vi "ReadFilesInFolder.vi"(7 "Numeric":i32, 8 "error in (no error)":errorcluster, 9 "Read entire Folder":bool, 10 "path":path, 11 "Path in":refnum<vi>) -> (0 "error out":errorcluster, 2 "t":i32, 3 "filenames":string[](array[string]))   [LabVIEW 2020]
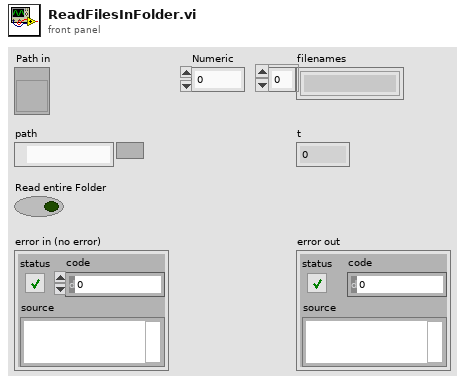
[diagram p1: front panel]
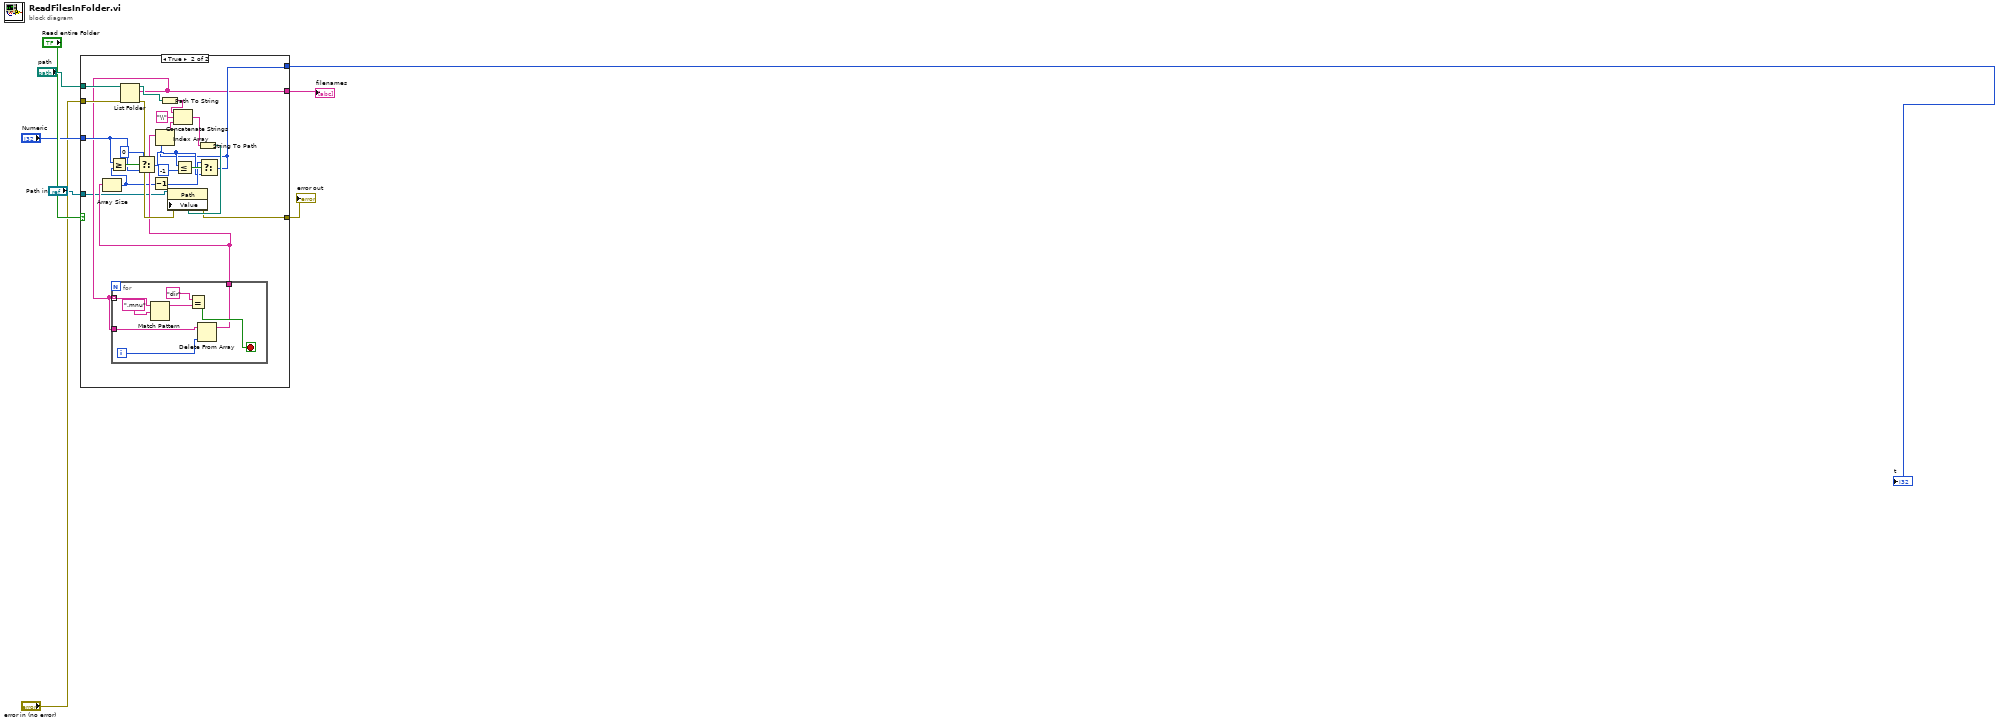
[diagram p0: block diagram]
diagram:
  n1 = case shown="True" "Read entire Folder" {
    tunnel: "error in (no error)" -> [w9 w26]
    tunnel: "Numeric" -> [w10 w24]
    tunnel: [w10 w15] -> w4
    tunnel: [w9 w14] -> w5
    tunnel: "path" -> [_ w13]
    tunnel: [_ w12] -> w8
    tunnel: "Path in" -> [_ w11]
    frame False {
    }
    frame True {
      n2 = List Folder(path=w13, error in=w26) -> (path out=w32:path, filenames=w12:string[], error out=w29:errorcluster)  [unwired: 2 in, 1 out]
      n3 = for {
        tunnel: w12 -> [w40] mode=indexing
        tunnel: w12 -> [w37]
        tunnel: [w33] -> w21
        i -> [w38]
        stop <- w34 stop-if-true
        n4 = Match Pattern(string=w40, regular expression=".mnu" ("string")) -> (before substring=w35:string)  [unwired: 1 in, 3 out]
        n5 = Equal?(x="dir" ("string"), y=w35) -> (x = y?=w34:bool)
        n6 = Delete From Array(array=w37, index=w38) -> (array with subset deleted=w33:string[])  [unwired: 1 in, 1 out]
      }
      n7 = Array Size(array=w21) -> (size(s)=w18:i32)
      n8 = Greater Or Equal?(x=w24, y=w18) -> (x >= y?=w25:bool)
      n9 = Select(t=0, s=w25, f=w24) -> (s? t:f=w16:i32)
      n10 = Decrement(x=w18) -> (x-1=w17:i32)
      n11 = Path To String(path=w32) -> (string=w31:string)
      n12 = Less Or Equal?(x=w16, y=-1) -> (x <= y?=w19:bool)
      n13 = Select(t=w17, s=w19, f=w16) -> (s? t:f=w15:i32)
      n14 = Index Array(array=w21, index=w15) -> (element=w22:string)
      n15 = Concatenate Strings(w31, "\\" ("string"), w22) -> (w30:string)
      n16 = String To Path(string=w30) -> (path=w28:path)
      n17 = property on="Property Node" class="Path"(reference=w11, error in=w29, "Value"=w28) -> (error out=w14:errorcluster)  [unwired: 1 out]
    }
  }
  "filenames" <- w8
  "error out" <- w5
  "t" <- w4
